vi "Limit Change.vi"(8 "error in (no error)":errorcluster, 10 "Limit Change":cluster{"Upper Limit":u8, "Lower Limit":u8}, 11 "Digital Acquisition in":refnum<class "Digital Acquisition.lvclass">) -> (0 "error out":errorcluster, 3 "Digital Acquisition out":refnum<class "Digital Acquisition.lvclass">)   [LabVIEW 2020, in "Digital Acquisition.lvlib" / "Digital Acquisition.lvclass"]
uses:
  Digital Acquisition.lvclass
  Digital Acquisition.lvclass/Digital Acquisition.ctl
  Counter/Counter Messages/Limits Change Msg/Limits Change Msg.lvclass/Limits Change Msg.ctl
  <vilib>/ActorFramework/Message Enqueuer/Message Enqueuer.lvclass/Message Enqueuer.ctl
  <vilib>/ActorFramework/Message Enqueuer/Enqueue.vi
  Counter/Counter Messages/Limits Change Msg/Limits Change Msg.lvclass
  C:/Program Files (x86)/National Instruments/LabVIEW 2020/vi.lib/ActorFramework/Message/Message.lvclass
  <vilib>/ActorFramework/Message Priority Queue/Priority Enqueue.vi
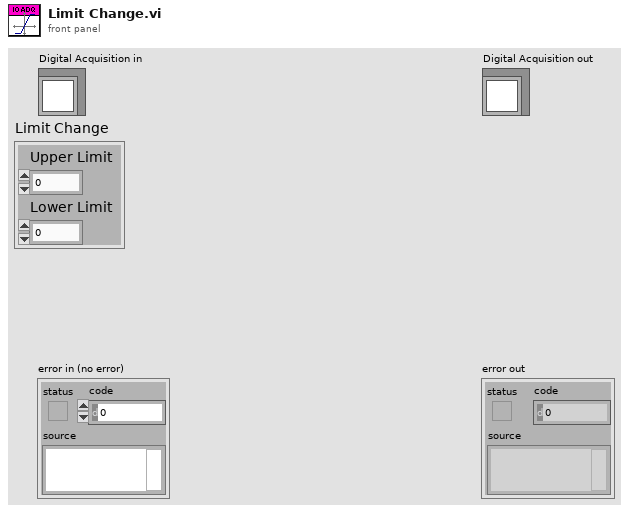
[diagram p1: front panel]
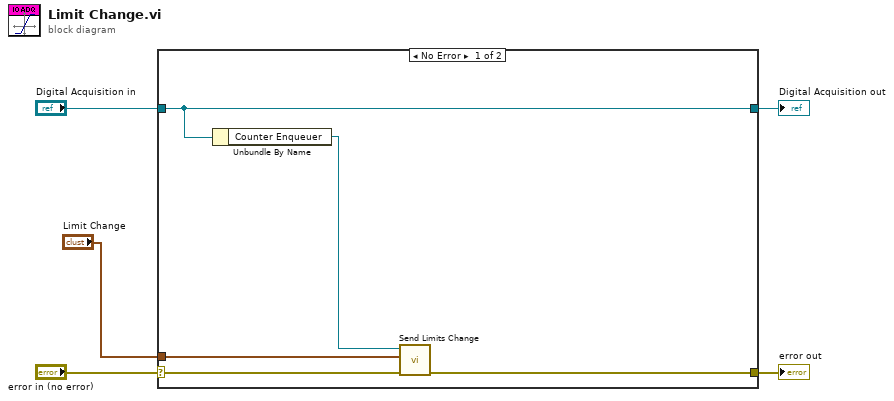
[diagram p0: block diagram]
diagram:
  n1 = case shown="No Error" "error in (no error)" {
    selector: "error in (no error)" -> [w10 w12]
    tunnel: [w9 w12] -> w4
    tunnel: [w8 w11] -> w2
    tunnel: "Digital Acquisition in" -> [w8 w11]
    tunnel: "Limit Change" -> [w6 _]
    frame No Error {
      n2 = Unbundle By Name(w8) -> ("Counter Enqueuer"=w7:refnum<class "Message Enqueuer.lvclass">)
      n3 = call "Send Limits Change.vi"("error in (no error)"=w10, "Limit Change"=w6, "Message Enqueuer"=w7) -> ("error out"=w9:errorcluster)  [unwired: 7 in, 1 out]
    }
    frame Error {
    }
  }
  "error out" <- w4
  "Digital Acquisition out" <- w2
